vi "Rx Streaming (Four Channels) (Host).vi"() -> ()   [LabVIEW 2020]
doc: "This template is for the Simple NI-USRP Streaming design, a design that shows the basics of streaming data from an NI 294x/295x device. Refer to the block diagram for more information about how to use this template."
uses:
  SubVIs/Start Trigger.ctl
  <vilib>/userdefined/Silver/nirio_resource_slv.ctl
  <vilib>/Utility/error.llb/DialogType.ctl
  SubVIs/Streaming Xvcr FPGA Ref.ctl
  <vilib>/Utility/error.llb/Error Cluster From Error Code.vi
  <vilib>/rvi/errors/niLvFpgaAdjustHostInterfaceError.vi
  <vilib>/measure/maspectr.llb/FFT Power Spectrum and PSD for 1 Chan (CDB).vi
  <vilib>/rvi/interface/nirviReadWriteControl/nirviReadWriteControl.xnode
  <vilib>/measure/NI_MAPro.lvlib
  NiFpgaLv.dll
  <vilib>/rvi/interface/Simulation/niFpgaSimulationCallBeginRW.vi
panel:
  out "packet start number":u32
  in  "experiment name":string="01_90_01"
  in  "number of packets to detect":u32=1
  out "csi are written":bool
  in  "trigger to write csi":bool
  out "samples are written":bool
  out "samples num":u32
  out "csi num":u32
  out "csi":string
  in  "trigger to write samples":bool
  out "samples":string
  out "subcarrier index":fxp<+/-,9,9>
  out "channel estimate valid":bool
  out "channel estimate":T1
  in  "configuration":T2={"primary channel selector"=0.25, "last OFDM symbol index"=10, "switch format detection states"=FALSE, "format"=enum."VHT", "bandwidth"=enum."80MHz"}
  in  "fifo 3 enable":bool
  in  "fifo 2 enable":bool
  in  "fifo 1 enable":bool
  in  "fifo 0 enable":bool
  out "RF to RX FIFO error out":errorcluster
  out "rx.parameters 2":T3={"rx.trigger select"=enum."Software", "rx.trigger enable"=FALSE, "rx.trigger sync enable"=FALSE, "rx.stream enable"=[FALSE, FALSE, FALSE, FALSE], "rx.software trigger"=FALSE, "rx.reset"=FALSE, "rx.abort"=FALSE, "rx.samples to acquire"=0, "rx.data sink"=enum."SFP Port 0", "rx.ddc parameters"=[{"output sample rate"=0.0, "delay"=0.0, "frequency shift"=0.0, "impairments"={"inline gain I"=0.0, "inline gain Q"=0.0, "cross gain I"=0.0, "cross gain Q"=0.0, "pre-gain offset I"=0.0, "pre-gain offset Q"=0.0, "post-gain offset I"=0.0, "post-gain offset Q"=0.0}, "phase"=0.0, "if frequency shift"=0.0}, {"output sample rate"=0.0, "delay"=0.0, "frequency shift"=0.0, "impairments"={"inline gain I"=0.0, "inline gain Q"=0.0, "cross gain I"=0.0, "cross gain Q"=0.0, "pre-gain offset I"=0.0, "pre-gain offset Q"=0.0, "post-gain offset I"=0.0, "post-gain offset Q"=0.0}, "phase"=0.0, "if frequency shift"=0.0}, {"output sample rate"=0.0, "delay"=0.0, "frequency shift"=0.0, "impairments"={"inline gain I"=0.0, "inline gain Q"=0.0, "cross gain I"=0.0, "cross gain Q"=0.0, "pre-gain offset I"=0.0, "pre-gain offset Q"=0.0, "post-gain offset I"=0.0, "post-gain offset Q"=0.0}, "phase"=0.0, "if frequency shift"=0.0}, {"output sample rate"=0.0, "delay"=0.0, "frequency shift"=0.0, "impairments"={"inline gain I"=0.0, "inline gain Q"=0.0, "cross gain I"=0.0, "cross gain Q"=0.0, "pre-gain offset I"=0.0, "pre-gain offset Q"=0.0, "post-gain offset I"=0.0, "post-gain offset Q"=0.0}, "phase"=0.0, "if frequency shift"=0.0}]}
  out "sample after sync":T4
  out "sample after sync valid":bool
  out "packet start":bool
  out "packet detected":bool
  out "sample num":i16
  in  "for filter":enum16{"20MHz", "40MHz"}(ring)
  in  "for shift":T5(ring)=enum."10MHz"
  out "was packet start true?":bool
  out "was packet detected true?":bool
  out "Imag":fxp<+/-,16,3>
  out "Real":fxp<+/-,16,3>
  out "lol":bool
  in  "kek":bool
  in  "rx config":T7={"transfer mode"=enum."Finite", "sample rate"=80000000.0, "number of samples"=8192, "start trigger"=enum."Immediate", "daughterboard 0 config"={"rf enable 0"=TRUE, "rf config 0"={"antenna"="RX1", "frequency"=2475000000.0, "gain"=40.0}, "rf enable 1"=TRUE, "rf config 1"={"antenna"="RX2", "frequency"=2475000000.0, "gain"=40.0}, "lo configuration"=enum."Shared"}, "daughterboard 1 config"={"rf enable 2"=TRUE, "rf config 2"={"antenna"="RX1", "frequency"=2475000000.0, "gain"=40.0}, "rf enable 3"=TRUE, "rf config 3"={"antenna"="RX2", "frequency"=2475000000.0, "gain"=40.0}, "lo configuration"=enum."Shared"}} {"daughterboard 1 config"."rf config 3"."gain" format="%#.1f"; "daughterboard 1 config"."rf config 3"."frequency" format="%#.3pHz"; "daughterboard 1 config"."rf config 2"."gain" format="%#.1f"; "daughterboard 1 config"."rf config 2"."frequency" format="%#.3pHz"; "daughterboard 0 config"."rf config 1"."gain" format="%#.1f"; "daughterboard 0 config"."rf config 1"."frequency" format="%#.3pHz"; "daughterboard 0 config"."rf config 0"."gain" format="%#.1f"; "daughterboard 0 config"."rf config 0"."frequency" format="%#.3pHz"; "sample rate" format="%#.3pS/s"}
  out "acquiring":bool caption="Acquiring"
  in  "USRP RIO device":T8="RIO0" caption="USRP RIO Device"
  in  "reference frequency source":string(combo)="Internal" caption="Reference Frequency Source"
  in  "indicator tab":T9(tab)
  out "power spectrum":cluster{"f0":dbl, "df":dbl, "magnitude":dbl[]}[](graph) caption="Power Spectrum"
  out "iq data":waveform(dbl)[](graph) caption="I & Q Data"
  out "rx.coerced config":T10 caption="Coerced Configurations" {"channel 3"."sample rate" format="%#.3pS/s"; "channel 3"."gain" format="%#_1f"; "channel 3"."if2 lo" format="%#.3pHz"; "channel 3"."if1 lo" format="%#.3pHz"; "channel 3"."frequency" format="%#.3pHz"; "channel 2"."sample rate" format="%#.3pS/s"; "channel 2"."gain" format="%#_1f"; "channel 2"."if2 lo" format="%#.3pHz"; "channel 2"."if1 lo" format="%#.3pHz"; "channel 2"."frequency" format="%#.3pHz"; "channel 1"."sample rate" format="%#.3pS/s"; "channel 1"."gain" format="%#_1f"; "channel 1"."if2 lo" format="%#.3pHz"; "channel 1"."if1 lo" format="%#.3pHz"; "channel 1"."frequency" format="%#.3pHz"; "channel 0"."sample rate" format="%#.3pS/s"; "channel 0"."gain" format="%#_1f"; "channel 0"."if2 lo" format="%#.3pHz"; "channel 0"."if1 lo" format="%#.3pHz"; "channel 0"."frequency" format="%#.3pHz"}
  in  "rx.stop":bool
  # "This template shows the basics of streaming data on a USRP-2945/2955 device. Open the Project Documentation folder of the sample project and select Simple NI-USRP Streaming 2945 2955.html for information about using LO sharing with this template."
  # "fpga to host fifo\nfor creating plots"
  # "from RF"
  # "Simple Rx Streaming"
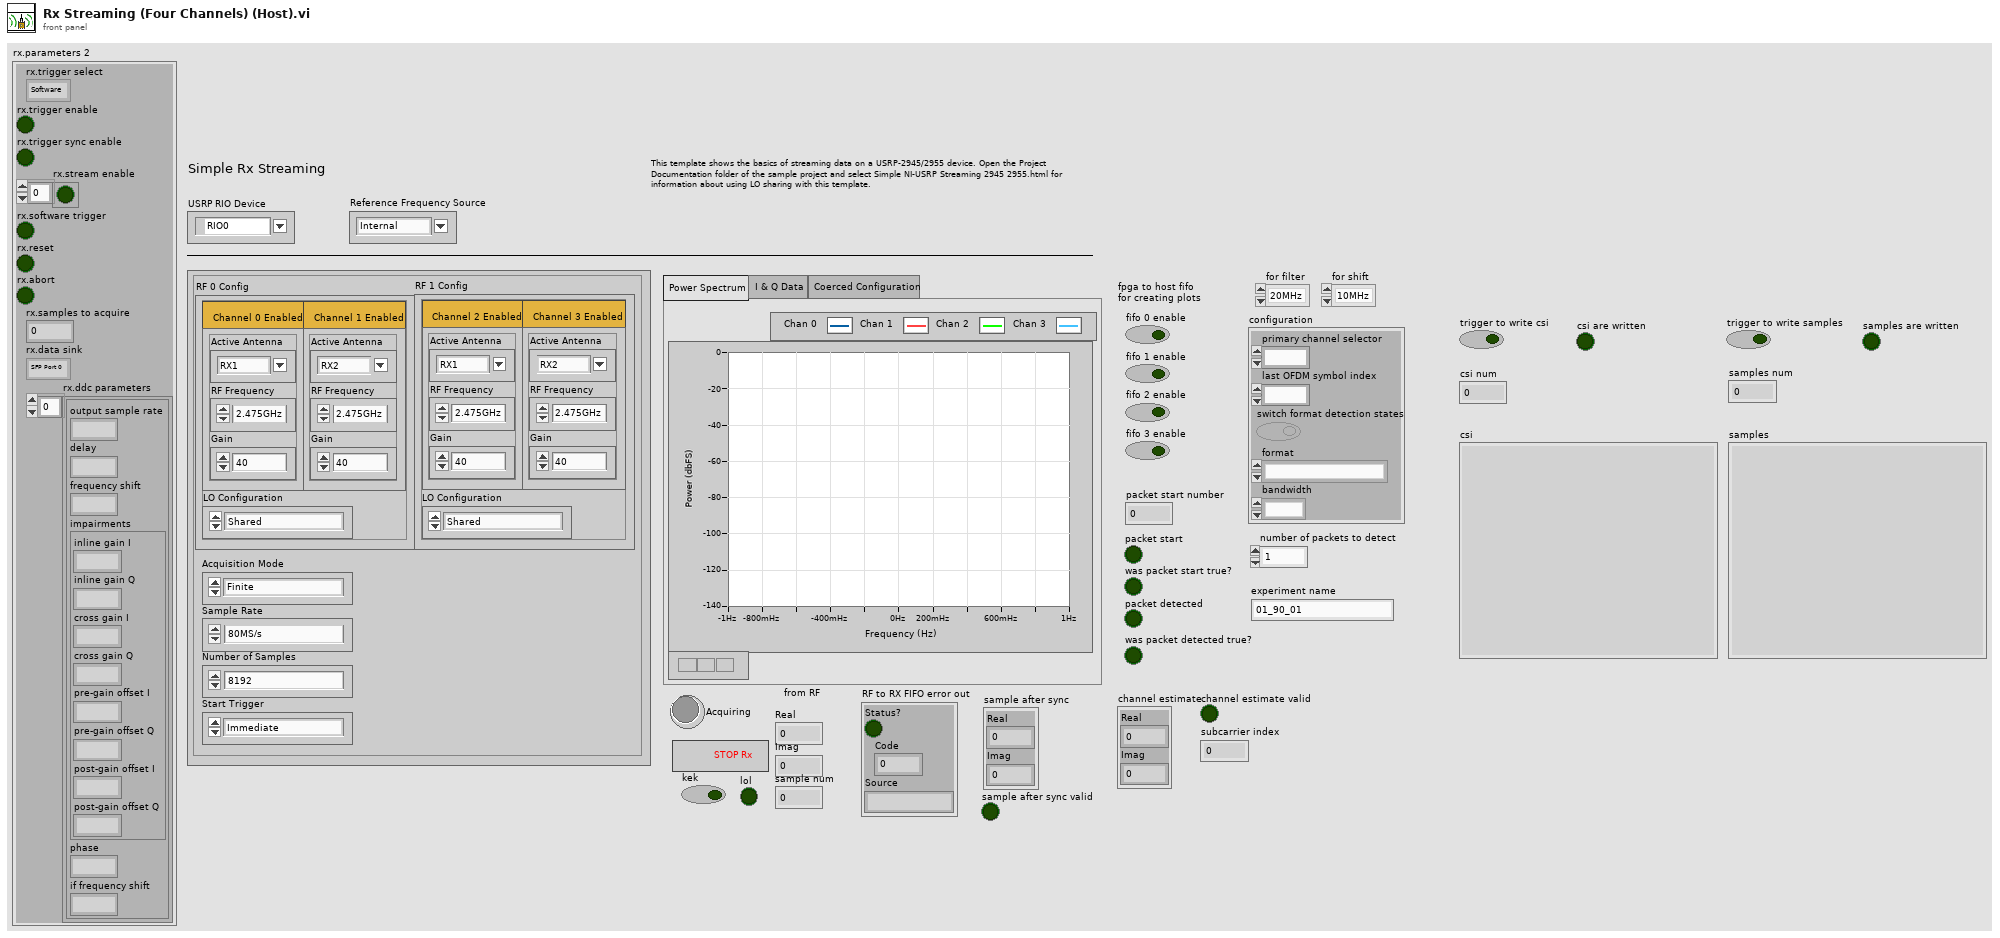
[diagram p1: front panel]
types:
  T1 = cluster{"Real":fxp<+/-,25,4>, "Imag":fxp<+/-,25,4>}
  T2 = cluster{"primary channel selector":fxp<+,2,0>, "last OFDM symbol index":u16, "switch format detection states":bool, "format":enum16{"NON_HT_OFDM", "VHT", "NON_HT_DUP_OFDM"}, "bandwidth":enum16{"20MHz", "40MHz", "80MHz"}}
  T3 = cluster{"rx.trigger select":enum8{"Software", "Digital Edge", "Rx Start Trigger", "Tx Start Trigger", "Immediate", "Future Time Event"}, "rx.trigger enable":bool, "rx.trigger sync enable":bool, "rx.stream enable":bool[], "rx.software trigger":bool, "rx.reset":bool, "rx.abort":bool, "rx.samples to acquire":u32, "rx.data sink":enum16{"SFP Port 0", "SFP Port 1", "Host"}, "rx.ddc parameters":cluster{"output sample rate":fxp<+,48,1>, "delay":fxp<+/-,16,0>, "frequency shift":fxp<+/-,48,0>, "impairments":cluster{"inline gain I":fxp<+/-,18,1>, "inline gain Q":fxp<+/-,18,1>, "cross gain I":fxp<+/-,18,1>, "cross gain Q":fxp<+/-,18,1>, "pre-gain offset I":fxp<+/-,18,1>, "pre-gain offset Q":fxp<+/-,18,1>, "post-gain offset I":fxp<+/-,18,1>, "post-gain offset Q":fxp<+/-,18,1>}, "phase":fxp<+/-,21,0>, "if frequency shift":fxp<+/-,48,0>}[]}
  T4 = cluster{"Real":fxp<+/-,16,3>, "Imag":fxp<+/-,16,3>}
  T5 = enum16{"-30MHz", "-20MHz", "-10MHz", "0MHz", "10MHz", "20MHz", "30MHz"}
  T6 = typedef "Start Trigger.ctl" = enum8{"Software", "Digital Edge", "Rx Start Trigger", "Tx Start Trigger", "Immediate", "Future Time Event"}
  T7 = cluster{"transfer mode":enum16{"Finite", "Continuous"}, "sample rate":dbl, "number of samples":u32, "start trigger":T6, "daughterboard 0 config":cluster{"rf enable 0":bool, "rf config 0":cluster{"antenna":string, "frequency":dbl, "gain":dbl}, "rf enable 1":bool, "rf config 1":cluster{"antenna":string, "frequency":dbl, "gain":dbl}, "lo configuration":enum16{"Independent", "Import", "Shared and Export", "Reimport", "Shared"}}, "daughterboard 1 config":cluster{"rf enable 2":bool, "rf config 2":cluster{"antenna":string, "frequency":dbl, "gain":dbl}, "rf enable 3":bool, "rf config 3":cluster{"antenna":string, "frequency":dbl, "gain":dbl}, "lo configuration":enum16{"Independent", "Import", "Shared and Export", "Reimport", "Shared"}}}
  T8 = typedef "nirio_resource_slv.ctl" = tag
  T9 = enum32{"Power Spectrum", "I & Q Data", "Coerced Configuration"}
  T10 = cluster{"channel 0":cluster{"frequency":dbl, "if1 lo":dbl, "if2 lo":dbl, "gain":dbl, "sample rate":dbl}[], "channel 1":cluster{"frequency":dbl, "if1 lo":dbl, "if2 lo":dbl, "gain":dbl, "sample rate":dbl}[], "channel 2":cluster{"frequency":dbl, "if1 lo":dbl, "if2 lo":dbl, "gain":dbl, "sample rate":dbl}[], "channel 3":cluster{"frequency":dbl, "if1 lo":dbl, "if2 lo":dbl, "gain":dbl, "sample rate":dbl}[], "device id":i32}
  T11 = typedef "DialogType.ctl" = u16
  T12 = typedef "Rx Channels.ctl" = cluster{"rx config":cluster{"channel configuration":cluster{"channel enable":bool, "channel configuration":cluster{"antenna":string, "frequency":dbl, "lo frequency":dbl, "level":dbl}}[], "transfer mode":enum16{"Finite", "Continuous"}, "sample rate":dbl, "number of samples":u32, "start trigger":T6}, "reference frequency source":string, "rx.data sink":enum16{"SFP Port 0", "SFP Port 1", "Host"}, "rx.enabled channels":string[], "vertical range":dbl[], "rx.coerced configurations":cluster{"coerced frequencies":dbl[], "coerced lo frequencies":dbl[], "coerced levels":dbl[], "coerced sample rates":dbl[]}}
  T13 = typedef "niUsrpRio Config v1 Host.lvlib/niUsrpRio Session.ctl" = cluster{"FPGA Interface":refnum<k20>, "RIO Interface Number":u32, "Data Clock Rate":u32, "FPGA Data Clock Rate":u32, "Global Settings Register Bus":T14, "Radio 0 Settings Register Bus":T14, "Radio 1 Settings Register Bus":T14, "Radio Settings Bus Semaphore":T15, "DB Queues":T16[], "Characterization Data Valid?":bool, "EEPROM Header":T17, "Device Data Header":T18, "EEPROM Characterization Header":T19, "Characterization Data":T20[], "FPGA Current Version":u32, "FPGA Oldest Compatible Version":u32, "Fixed Logic Current Version":u32, "Fixed Logic Oldest Compatible Version":u32, "FPGA Radio Settings Bus Current Version":u32, "FPGA Radio Settings Bus Oldest Compatible Version":u32, "FPGA Board Config Current Version":u32, "FPGA Board Config Oldest Compatible Version":u32, "Daughterboard Clock Rate":u32, "daughterboard configuration session handles":u64[]}
  T14 = typedef "niInstr Register Bus v0 Host.lvlib/Register Bus Session.ctl" = refnum<queue>
  T15 = typedef "Semaphore RefNum" = refnum<k1>
  T16 = typedef "niUsrpRio Config v1 Host.lvlib/DB Queue Reference.ctl" = refnum<queue>
  T17 = typedef "niUsrpRio Config v1 Host.lvlib/EEPROM Header.ctl" = cluster{"Checksum":u32, "Product Code":u16, "Hardware Current Version":u16, "Hardware Oldest Compatible Version":u16, "EEPROM Map Current Version":u16, "EEPROM Map Oldest Compatible Version":u16, "User Password":string, "Pointer to Factory Header":u32, "Pointer to User Header":u32, "Recommended Interval":u16, "Number of Reserved Bytes":i32, "Number of Daughterboards":u8, "Daughterboard IDs":u16[], "Daughterboard Serial Numbers":string[]}
  T18 = typedef "niUsrpRio Config v1 Host.lvlib/EEPROM Device Data Header.ctl" = cluster{"Checksum":u32, "Number of Channels":u8, "Number of Gain Settings":u16[], "Pointer to Characterization Data":u32[], "Number of Reserved Bytes":i32, "Number of Frequencies":u16[]}
  T19 = typedef "niUsrpRio Config v1 Host.lvlib/EEPROM Characterization Header.ctl" = cluster{"Checksum":u32, "Date":timestamp, "Temperature":sgl, "Misc. Info":string, "Pointer to Device Data Header":u32, "Number of Reserved Bytes":i32}
  T20 = typedef "niUsrpRio Config v1 Host.lvlib/Characterization Data.ctl" = cluster{"Gains[dB]":dbl[], "Frequencies [Hz]":dbl[], "IQ Imbalance Table":T21[], "Measured Gains[dB]":dbl[][]}
  T21 = typedef "niUsrpRio Config v1 Host.lvlib/IQ Imbalance.ctl" = cluster{"Gain Imbalance [linear]":dbl, "Phase Imbalance [radians]":dbl, "Offset":cdb}
  T22 = cluster{"coerced frequencies":dbl[], "coerced if1 frequencies":dbl[], "coerced if2 frequencies":dbl[], "coerced gain":dbl[], "coerced sample rates":dbl[]}
  T23 = typedef "Streaming Xvcr FPGA Ref.ctl" = refnum<k20>
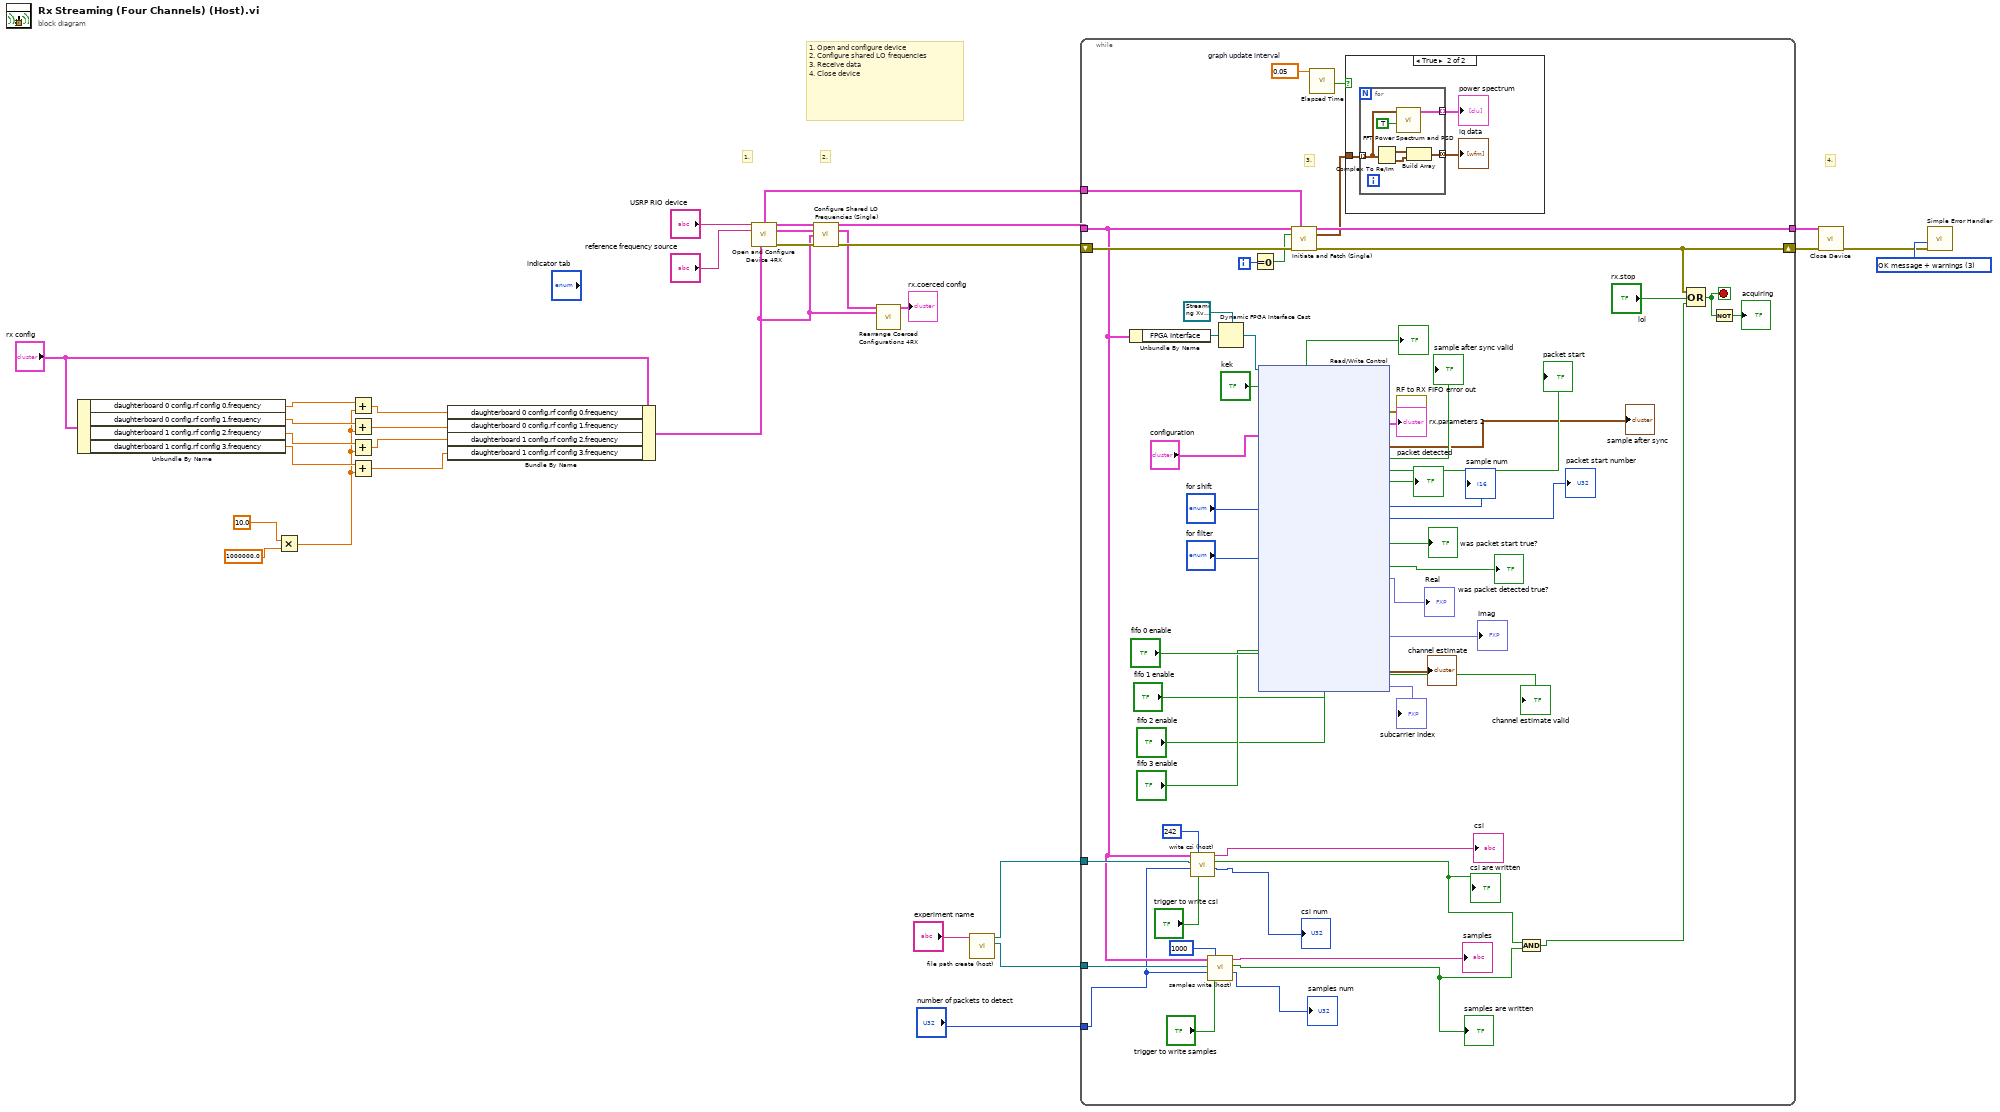
[diagram p0: block diagram]
diagram:
  w31 = T11 3 items=["no dialog", "OK message", "continue or stop message", "OK message + warnings", "continue/stop + warnings"] ("type of dialog (OK msg:1)")
  # "2."
  # "4."
  # "1. Open and configure device\n2. Configure shared LO frequencies\n3. Receive data\n4. Close device"
  # "1."
  n1 = Unbundle By Name("rx config") -> ("daughterboard 0 config.rf config 0.frequency"=w13:dbl, "daughterboard 0 config.rf config 1.frequency"=w12:dbl, "daughterboard 1 config.rf config 2.frequency"=w11:dbl, "daughterboard 1 config.rf config 3.frequency"=w10:dbl)
  n2 = Multiply(x=10.0 ("daughterboard 1 config.rf config 3.frequency"), y=1000000.0) -> (x*y=w5:dbl)
  n3 = Add(x=w13, y=w5) -> (x+y=w17:dbl)
  n4 = Add(x=w12, y=w5) -> (x+y=w14:dbl)
  n5 = Add(x=w11, y=w5) -> (x+y=w15:dbl)
  n6 = Add(x=w10, y=w5) -> (x+y=w16:dbl)
  n7 = Bundle By Name(cluster="rx config", "daughterboard 0 config.rf config 0.frequency"=w17, "daughterboard 0 config.rf config 1.frequency"=w14, "daughterboard 1 config.rf config 2.frequency"=w15, "daughterboard 1 config.rf config 3.frequency"=w16) -> (w8:T7)
  n8 = call "Open and Configure Device 4RX.vi"("USRP RIO Device"="USRP RIO device", "reference frequency source"="reference frequency source", "rx config"=w8) -> ("rx channels"=w25:T12, "niUsrpRio Session (out)"=w23:T13, "rx.coerced configurations"=w20:T22, "error out"=w21:errorcluster)  [unwired: 9 in]
  n9 = call "Configure Shared LO Frequencies (Single).vi"("niUsrpRio Session"=w23, "rx.coerced config"=w20, "rx config"=w8, "error in"=w21) -> ("niUsrpRio Session (out)"=w18:T13, "rx.coerced config out"=w19:T22, "error out"=w22:errorcluster)  [unwired: 9 in]
  n10 = call "Rearrange Coerced Configurations 4RX.vi"("rx.coerced configurations"=w19, "rx config"=w8) -> ("coerced configurations"=→"rx.coerced config":T10)  [unwired: 13 in]
  n11 = call "file path create (host).vi"("experiment name"="experiment name") -> ("samples file"=w2:refnum<file>, "csi file"=w3:refnum<file>)  [unwired: 8 in, 1 out]
  n12 = while {
    tunnel: w18 -> [w34]
    tunnel: [w81] -> w26
    tunnel: w25 -> [w78]
    shift-right: [w82] -> w27
    shift-left: w22 -> [w84]
    tunnel: w3 -> [w44]
    tunnel: w2 -> [w33]
    tunnel: "number of packets to detect" -> [w32]
    i -> [w83]
    stop <- w79 stop-if-true
    w76 = 0.05  # graph update interval
    # "3."
    # "Acquire and Fetch a waveform"
    n13 = Unbundle By Name(w34) -> ("FPGA Interface"=w48:refnum<k20>)
    n14 = call "write csi (host).vi"("trigger to write csi"="trigger to write csi", "csi num"=u32 242 ("csi per packet"), "number of packets to detect"=w32, "file ref"=w44, "fpga cluster"=w34) -> ("csi num"=→"csi num":u32, "csi is written"=w41:bool, "csi"=→"csi":string)  [unwired: 4 in]
    "csi are written" <- w41
    n15 = call "samples write (host).vi"("trigger to write samples"="trigger to write samples", "samples num"=u32 1000 ("samples per packet"), "number of packets to detect"=w32, "file for writing samples"=w33, "fpga cluster"=w34) -> ("samples num"=→"samples num":u32, "samples is written"=w36:bool, "samples"=→"samples":string)  [unwired: 4 in]
    "samples are written" <- w36
    n16 = Dynamic FPGA Interface Cast(Session In=T23 refnum ("Type"), Type=w48) -> (Session Out=w46:T23)
    n17 = Equal To 0?(x=w83) -> (x = 0?=w75:bool)
    n18 = xnode "Read/Write Control"("FPGA VI Reference In"=w46, "kek"="kek", "configuration"="configuration", "for shift"="for shift", "for filter"="for filter", "fifo 0 enable"="fifo 0 enable", "fifo 1 enable"="fifo 1 enable", "fifo 2 enable"="fifo 2 enable", "fifo 3 enable"="fifo 3 enable") -> ("lol"=→"lol":bool, "FIFO error out 2"=→"RF to RX FIFO error out":errorcluster, "rx.parameters 2"=→"rx.parameters 2":T3, "sample out"=→"sample after sync":T4, "sample out valid"=→"sample after sync valid":bool, "packet start"=→"packet start":bool, "packet detected"=→"packet detected":bool, "sample number"=→"sample num":i16, "packet start number"=→"packet start number":u32, "was packet start true?"=→"was packet start true?":bool, "was packet detected true? 2"=→"was packet detected true?":bool, "Real"=→"Real":fxp<+/-,16,3>, "Imag"=→"Imag":fxp<+/-,16,3>, "channel estimate"=→"channel estimate":T1, "channel estimate valid"=→"channel estimate valid":bool, "subcarrier index"=→"subcarrier index":fxp<+/-,9,9>)  [unwired: 1 in, 4 out]
    n19 = call "Initiate and Fetch (Single).vi"("niUsrpRio Session"=w34, "rx channels"=w78, "first iteration"=w75, "error in"=w84) -> ("niUsrpRio Session (out)"=w81:T13, "complex baseband data"=w72:waveform(cdb)[], "error out"=w82:errorcluster)  [unwired: 9 in]
    n20 = call "Elapsed Time"("Time Target (s)"=w76) -> ("Time has Elapsed"=w77:bool)  [unwired: 11 in, 7 out]
    n21 = case shown="True" w77 {
      tunnel: w72 -> [_ w88]
      frame False {
      }
      frame True {
        n22 = for {
          tunnel: [w92] -> w87 mode=concatenating
          tunnel: [w90] -> w86 mode=indexing
          tunnel: w88 -> [w91] mode=indexing
          n23 = Complex To Re/Im(x + iy=w91) -> (x=w94:waveform(dbl), y=w93:waveform(dbl))
          n24 = call-poly <vilib>:"FFT Power Spectrum and PSD.vi"("dB On (F)"=TRUE, "time signal"=w91) -> ("Power Spectrum / PSD"=w90:cluster{"f0":dbl, "df":dbl, "magnitude":dbl[]})  [unwired: 6 in, 3 out]
          n25 = Build Array(w94, w93) -> (w92:waveform(dbl)[])
        }
        "power spectrum" <- w86
        "iq data" <- w87
      }
    }
    n26 = And(x=w41, y=w36) -> (x .and. y?=w49:bool)
    n27 = Compound Arithmetic op=OR(w82, "rx.stop", w49) -> (w79:bool)
    n28 = Not(x=w79) -> (.not. x?=→"acquiring":bool)
  }
  n29 = call "Close Device.vi"("niUsrpRio Session"=w26, "error in"=w27) -> ("error out"=w30:errorcluster)  [unwired: 13 in]
  n30 = call <vilib>:"Simple Error Handler.vi"("type of dialog (OK msg:1)"=w31, "error in (no error)"=w30) -> ()  [unwired: 3 in, 5 out]
